vi "NB_WriteAttribute.vi"(8 "Error In":errorcluster, 11 "object in":refnum<class "NativeBaseTemplate_4x4x4.lvclass">) -> (0 "Error Out":errorcluster, 3 "object out":refnum<class "NativeBaseTemplate_4x4x4.lvclass">)   [LabVIEW 2020, in "NativeBaseTemplate_4x4x4.lvclass"]
uses:
  <resource>/Framework/Providers/Open_GDS/ClassProviders/Provider_LvNativeClass/Templates/NativeBaseTemplate_4x4x4/NativeBaseTemplate_4x4x4.lvclass
  <resource>/Framework/Providers/Open_GDS/ClassProviders/Provider_LvNativeClass/Templates/NativeBaseTemplate_4x4x4/NativeBaseTemplate_4x4x4.lvclass/NativeBaseTemplate_4x4x4.ctl
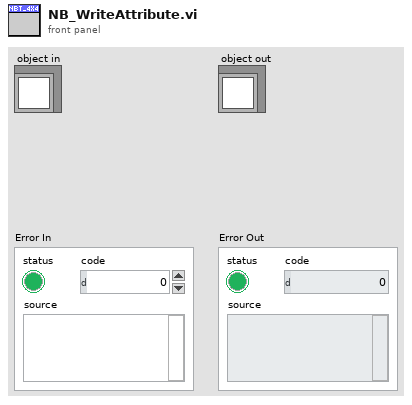
[diagram p1: front panel]
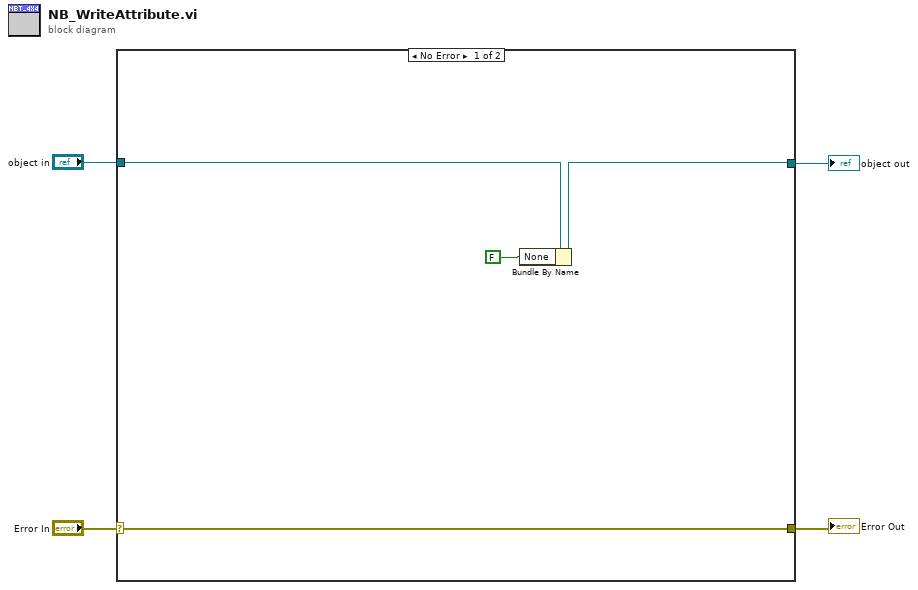
[diagram p0: block diagram]
diagram:
  n1 = case shown="No Error" "Error In" {
    selector: "Error In" -> [w8 w10]
    tunnel: [w8 w10] -> w3
    tunnel: [w6 w9] -> w1
    tunnel: "object in" -> [w7 w9]
    frame No Error {
      n2 = Bundle By Name(cluster=w7, "None"=FALSE) -> (w6:refnum<class "NativeBaseTemplate_4x4x4.lvclass">)
    }
    frame Error {
    }
  }
  "Error Out" <- w3
  "object out" <- w1
